vi "UpdateDestroyPosition.vi"(2 "AFM Mode":bool, 3 "Image Settings":T1 {"2nd Axis" items=["x", "y", "z"]; "1st Axis" items=["x", "y", "z"]; "Time Resolution\n(ms/pixel)" format="%.2f"; "Image Resolution (nm/pixel)"."z" format="%.2f"; "Image Resolution (nm/pixel)"."y" format="%.2f"; "Image Resolution (nm/pixel)"."x" format="%.2f"; "Image Size (µm)"."z" format="%.2f"; "Image Size (µm)"."y" format="%.2f"; "Image Size (µm)"."x" format="%.2f"; "End Position (µm)"."z" format="%.2f"; "End Position (µm)"."y" format="%.2f"; "End Position (µm)"."x" format="%.2f"; "Start Position (µm)"."z" format="%.2f"; "Start Position (µm)"."y" format="%.2f"; "Start Position (µm)"."x" format="%.2f"}) -> (1 "error out":errorcluster)   [LabVIEW 2009]
uses:
  ImageSettings.ctt
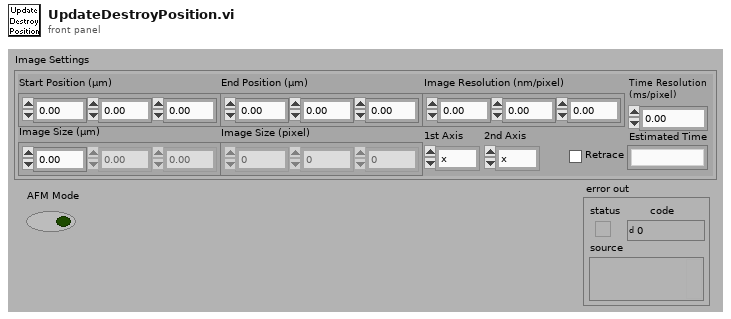
[diagram p1: front panel]
types:
  T1 = typedef "ImageSettings.ctt" = cluster{"Start Position (µm)":cluster{"x":dbl, "y":dbl, "z":dbl}, "End Position (µm)":cluster{"x":dbl, "y":dbl, "z":dbl}, "Image Resolution (nm/pixel)":cluster{"x":dbl, "y":dbl, "z":dbl}, "Image Size (µm)":cluster{"x":dbl, "y":dbl, "z":dbl}, "Image Size (pixel)":cluster{"x":u32, "y":u32, "z":u32}, "Time Resolution\n(ms/pixel)":dbl, "1st Axis":u16, "2nd Axis":u16, "Retrace":bool, "Estimated Time":string}
  T2 = typedef "PickImage.ctl" = cluster{"Rawdata":T3, "Mask":T3, "Display":T3, "Coefficients (2D)":sgl[][], "Destroy Index":u32}
  T3 = typedef "IMAQ Image.ctl" = refnum<image>
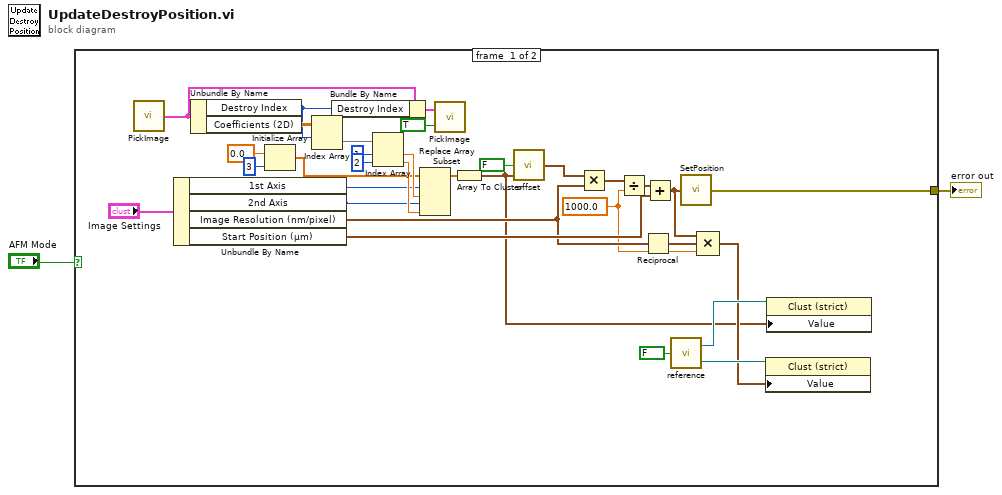
[diagram p0: block diagram]
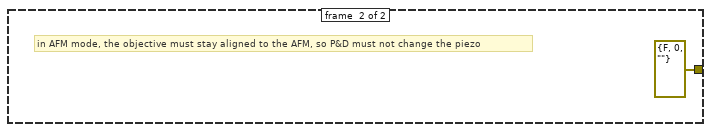
[diagram p2: hidden frame]
diagram:
  n1 = case shown="True" "AFM Mode" {
    tunnel: [w3 errorcluster {"status"=FALSE, "code"=0, "source"=""} ("error out")] -> w1
    frame #0 {
      w13 = 1000.0
      n2 = call "PickImage.vi"() -> ("Image (output)"=w19:T2)  [unwired: 2 in]
      n3 = Unbundle By Name("Image Settings") -> ("1st Axis"=w28:u16, "2nd Axis"=w29:u16, "Image Resolution (nm/pixel)"=w14:cluster{"x":dbl, "y":dbl, "z":dbl}, "Start Position (µm)"=w34:cluster{"x":dbl, "y":dbl, "z":dbl})
      n4 = Unbundle By Name(w19) -> ("Destroy Index"=w4:u32, "Coefficients (2D)"=w20:sgl[][])
      n5 = Initialize Array(0.0 ("element"), 3 ("dimension size")) -> (w27:dbl[])
      n6 = Index Array(array=w20, index (row)=w4) -> (element=w22:sgl[])  [unwired: 1 in]
      n7 = Bundle By Name(cluster=w19, "Destroy Index"=w4) -> (w18:T2)
      n8 = Index Array(array=w22, index #1=1 ("index"), index #2=2 ("index")) -> (element #1=w31:sgl, element #2=w32:sgl)
      n9 = Replace Array Subset(array=w27, new element #1=w31, index #1=w28, new element #2=w32, index #2=w29) -> (w30:dbl[])
      n10 = call "PickImage.vi"("Get/Set"=TRUE, "Images (input)"=w18) -> ()  [unwired: 1 out]
      n11 = Array To Cluster(array=w30) -> (cluster=w5:cluster{"[0]":dbl, "[1]":dbl, "[2]":dbl})
      n12 = call "offset.vi"("coordinates (in)"=w5, "set?"=FALSE) -> ("coordinates (out)"=w11:cluster{dbl, dbl, dbl})  [unwired: 1 in]
      n13 = Multiply(x=w11, y=w14) -> (x*y=w33:cluster{dbl, dbl, dbl})
      n14 = Divide(x=w33, y=w13) -> (x/y=w16:cluster{dbl, dbl, dbl})
      n15 = Reciprocal(x=w14) -> (1/x=w12:cluster{"x":dbl, "y":dbl, "z":dbl})
      n16 = Add(x=w16, y=w34) -> (x+y=w15:cluster{dbl, dbl, dbl})
      n17 = call "reference.vi"("set?"=FALSE) -> ("coordinates (pixel) 2"=w8:refnum<vi>, "Pickcoord. (pixel) 2"=w7:refnum<vi>)  [unwired: 3 in]
      n18 = call "SetPosition.vi"("Current Position (µm)"=w15) -> ("error out"=w3:errorcluster)
      n19 = Compound Arithmetic op=MULTIPLY(w15, w12, w13) -> (w6:cluster{dbl, dbl, dbl})
      n20 = property class="Clust (strict)"(reference=w8, "Value"=w6) -> ()  [unwired: 1 in, 2 out]
      n21 = property class="Clust (strict)"(reference=w7, "Value"=w5) -> ()  [unwired: 1 in, 2 out]
    }
    frame #1 {
      # "in AFM mode, the objective must stay aligned to the AFM, so P&D must not change the piezo"
    }
  }
  "error out" <- w1
